vi "Init Hardware.vi"(8 "error in (no error)":errorcluster, 11 "RP I-V Driver in":refnum<class "RP I-V Driver.lvclass">) -> (0 "error out":errorcluster, 3 "RP I-V Driver out":refnum<class "RP I-V Driver.lvclass">)   [LabVIEW 2018, in "RP I-V Driver.lvclass"]
uses:
  RP I-V Driver.lvclass
  C:/github/NHMFL_Core/Libraries/Red Pitaya/Red Pitaya Digitizer/Red Pitaya Digitizer.lvclass
  C:/github/NHMFL_Core/Libraries/Instruments/Pulse Driver/Pulse Driver.lvclass
  RP Command.ctl
  Red Pitaya Digitizer/Red Pitaya Digitizer.lvclass/Red Pitaya Digitizer.ctl
  RP I-V Driver.lvclass/RP I-V Driver.ctl
  Red Pitaya Digitizer/Read RP Instrument.vi
  Red Pitaya Digitizer/Write RP Instrument.vi
  Write Output waveform.vi
  Red Pitaya Digitizer/Red Pitaya Digitizer.lvclass
  RP Instrument/RP Instrument.lvclass
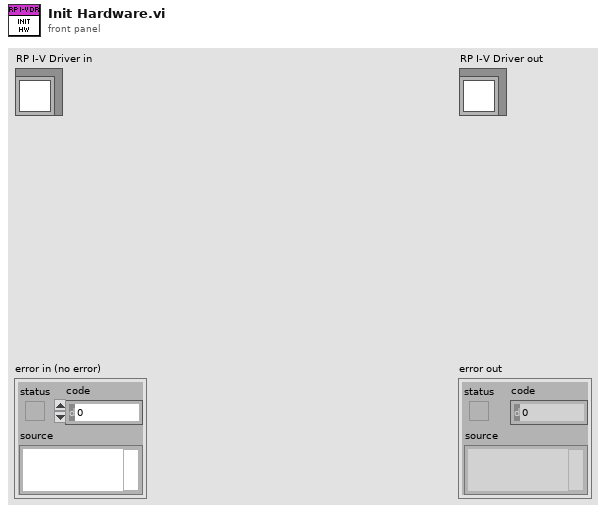
[diagram p1: front panel]
types:
  T1 = typedef "RP Command.ctl" = enum16{"Reset", "Read IDN", "Stop server", "Get status", "Get temperature", "Connect client", "Arm", "Software trigger", "Get whole buffer", "Get chunk", "System call", "Get config", "Set config", "Recieve data", "Recieve Calibartion", "Transmit data"}
  T2 = typedef "RP I-V Configuration.ctl" = cluster{"I-V parameters":T3, "Ranges":dbl[], "Pre-trigger duration":dbl, "Post-trigger duration":dbl, "Output delay":dbl}
  T3 = typedef "I-V parameters.ctl" = cluster{"Start magnitude":dbl, "Magnitude increment":dbl, "End magnitude":dbl, "Ramp length":i32, "Top  length":i32, "Threshold ":dbl, "Processing delay":u16, "Valhalla range":dbl, "Interpolation":i32, "Stop after":u16, "Detector window":i32}
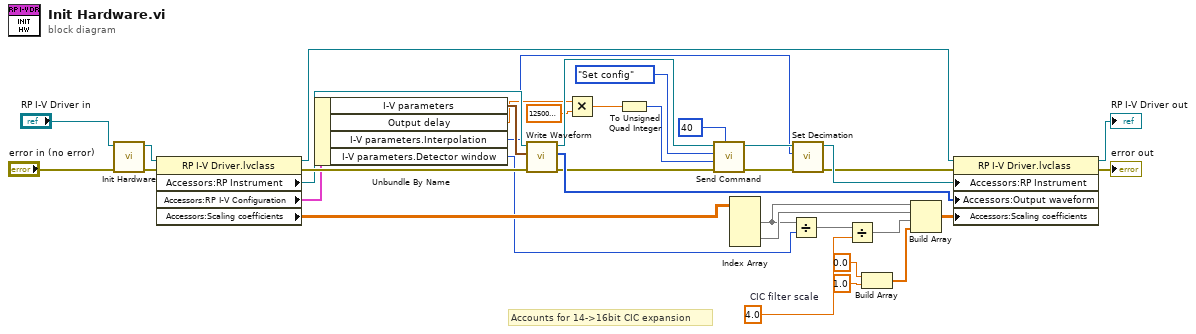
[diagram p0: block diagram]
diagram:
  w1 = 4.0  # CIC filter scale
  # "Accounts for 14->16bit CIC expansion"
  n1 = call-parent "Init Hardware.vi"("error in (no error)"="error in (no error)", "Red Pitaya Digitizer in"="RP I-V Driver in") -> ("error out"=w21:errorcluster, "Red Pitaya Digitizer out"=w20:refnum<class "RP I-V Driver.lvclass">)  [unwired: 8 in]
  n2 = property class="RP I-V Driver.lvclass"(reference=w20, error in=w21) -> (reference out=w36:refnum<class "RP I-V Driver.lvclass">, error out=w35:errorcluster, "Accessors:RP Instrument"=w34:refnum<class "RP Instrument.lvclass">, "Accessors:RP I-V Configuration"=w28:T2, "Accessors:Scaling coefficients"=w12:dbl[][])
  n3 = Unbundle By Name(w28) -> ("I-V parameters"=w27:T3, "Output delay"=w4:dbl, "I-V parameters.Interpolation"=w13:i32, "I-V parameters.Detector window"=w9:i32)
  n4 = call-dynamic "Write Waveform.vi"("error in (no error)"=w35, "I-V parameters"=w27, "RP Instrument in"=w34) -> ("error out"=w31:errorcluster, "Output Waveform"=w33:i16[], "RP Instrument out"=w32:refnum<class "RP Instrument.lvclass">)  [unwired: 6 in]
  n5 = Multiply(x=w4, y=125000000.0) -> (x*y=w25:dbl)
  n6 = To Unsigned Quad Integer(1:w25) -> (0:w24:u64)
  n7 = call-dynamic "Send Command.vi"("Config offset"=u64 40, "error in (no error)"=w31, "Command payload"=w24, "Command number"=RP_Command."Set config", "RP Instrument in"=w32) -> ("error out"=w15:errorcluster, "RP Instrument out"=w17:refnum<class "RP Instrument.lvclass">)  [unwired: 5 in]
  n8 = Index Array(array=w12) -> (element #1=w10:dbl[], element #2=w11:dbl[])  [unwired: 4 in]
  n9 = Divide(x=w10, y=w9) -> (x/y=w2:dbl[])
  n10 = call-dynamic "Set Decimation.vi"("error in (no error)"=w15, "Decimation"=w13, "RP Instrument in"=w17) -> ("error out"=w14:errorcluster, "RP Instrument out"=w16:refnum<class "RP Instrument.lvclass">)  [unwired: 7 in]
  n11 = Divide(x=w2, y=w1) -> (x/y=w3:dbl[])
  n12 = Build Array(0.0 ("element"), 1.0 ("element")) -> (w6:dbl[])
  n13 = Build Array(w10, w11, w3, w6) -> (w5:dbl[][])
  n14 = property class="RP I-V Driver.lvclass"(reference=w36, error in=w14, "Accessors:RP Instrument"=w16, "Accessors:Output waveform"=w33, "Accessors:Scaling coefficients"=w5) -> (reference out=→"RP I-V Driver out":refnum<class "RP I-V Driver.lvclass">, error out=→"error out":errorcluster)
